vi "Close Framework Event Log.vi"(8 "error in (no error)":errorcluster, 10 "Deferred Close Time (0 ms)":u32, 11 "IObserver in":refnum<class "IObserver.lvclass">) -> ()   [LabVIEW 2019, in "IObserver.lvlib" / "IObserver.lvclass"]
uses:
  <vilib>/gpm_packages/@cs/mva-core/Source/IObserver/IObserver/IObserver.lvclass
  <vilib>/gpm_packages/@cs/mva-core/Source/IObserver/IObserver/IObserver.lvclass/IObserver.ctl
  <vilib>/gpm_packages/@cs/event-logger/Source/Composed Log/LoggerReference/LoggerReference.lvclass
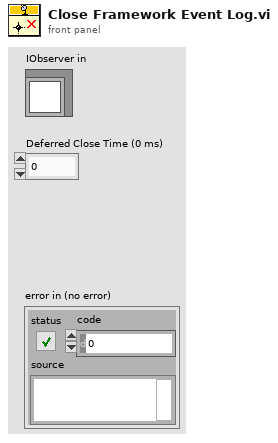
[diagram p1: front panel]
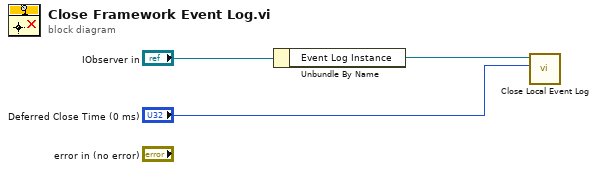
[diagram p0: block diagram]
diagram:
  n1 = Unbundle By Name("IObserver in") -> ("Event Log Instance"=w2:refnum<class "LoggerReference.lvclass">)
  n2 = call <vilib>:"Close Local Event Log.vi"("Deferred Close Time (0 ms)"="Deferred Close Time (0 ms)", "Log Instance"=w2) -> ()  [unwired: 9 in, 1 out]
